vi "Replace Children.vi"(8 "error in (no error)":errorcluster, 10 "New Children":refnum<class "Data Item.lvclass">[](array[class]), 11 "Reference in":refnum<class "Reference.lvclass">) -> (0 "error out":errorcluster, 3 "Reference out":refnum<class "Reference.lvclass">)   [LabVIEW 2018, in "VILab.lvlib" / "Reference.lvclass"]
uses:
  Reference.lvclass
  Data Item.lvclass
  Attribute.lvclass
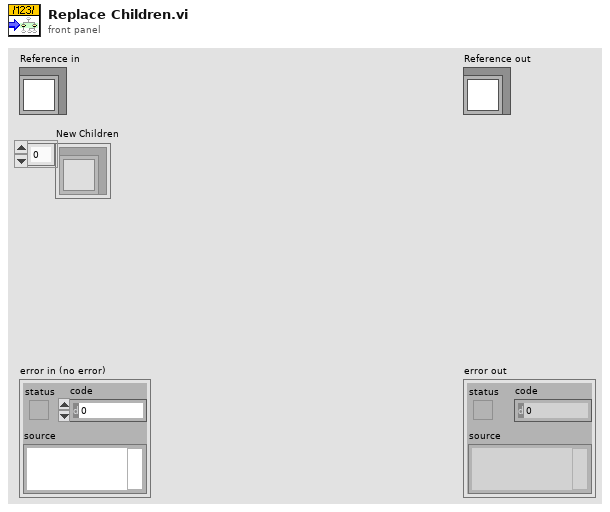
[diagram p1: front panel]
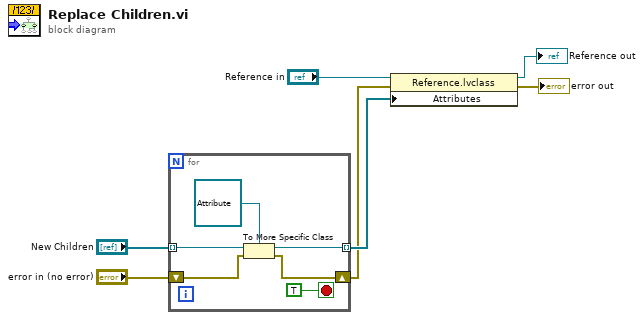
[diagram p0: block diagram]
diagram:
  n1 = for {
    tunnel: "New Children" -> [w13] mode=indexing
    tunnel: [w12] -> w5 mode=indexing
    shift-right: [w8] -> w3
    shift-left: "error in (no error)" -> [w9]
    stop <- TRUE stop-if-true
    n2 = To More Specific Class(target class=refnum<class "Attribute.lvclass"> refnum ("VILab.lvlib:Attribute.lvclass"), reference=w13, error in=w9) -> (specific class reference=w12:refnum<class "Attribute.lvclass">, error out=w8:errorcluster)
  }
  n3 = property class="Reference.lvclass"(reference="Reference in", error in=w3, "Attributes"=w5) -> (reference out=→"Reference out":refnum<class "Reference.lvclass">, error out=→"error out":errorcluster)
